vi "MOCON_get_rdg.vi"(4 "Channel Name":string, 7 "Address":T1={"Main"=57344, "Ch."=7, "Sub"=0, "Port Name"="10.245.69.44"}) -> (0 "Output":dbl format="%_5g", 3 "Status note":string)   [LabVIEW 2020]
uses:
  ADAM Client/Sub VIs/ADAM Controls/Address.ctl
  ADAM Client/Sub VIs/ADAM Controls/Remember_value_mode.ctl
panel:
  out "UDPopenError":errorcluster
  out "UDPreadError":errorcluster
  # "Channels:\n0: Timestamp\n1: \n2: \n3: Concentration\n4:\n5:\n6:\n7: Sample Flow\n8: Fuel Flow\n9: Air Flow\n10: Det. Curr.\n11:\n12:\n13: Temperature"
  # "Started life as ClimatronicsUDP_get_rdg.vi"
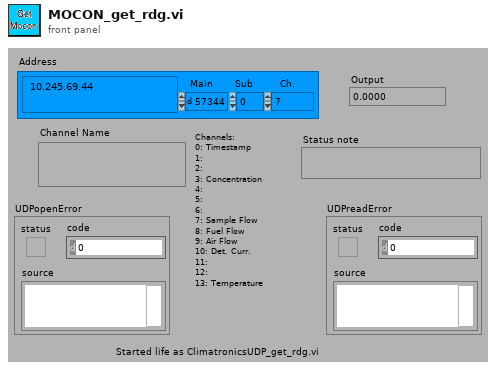
[diagram p1: front panel]
types:
  T1 = typedef "Address.ctl" = cluster{"Main":i32, "Ch.":i32, "Sub":i32, "Port Name":string}
  T2 = typedef "Remember_value_mode.ctl" = enum16{"Read only", "Read and Write"}
  T3 = enum16{"Standard", "Buffered", "CRLF", "Immediate"}
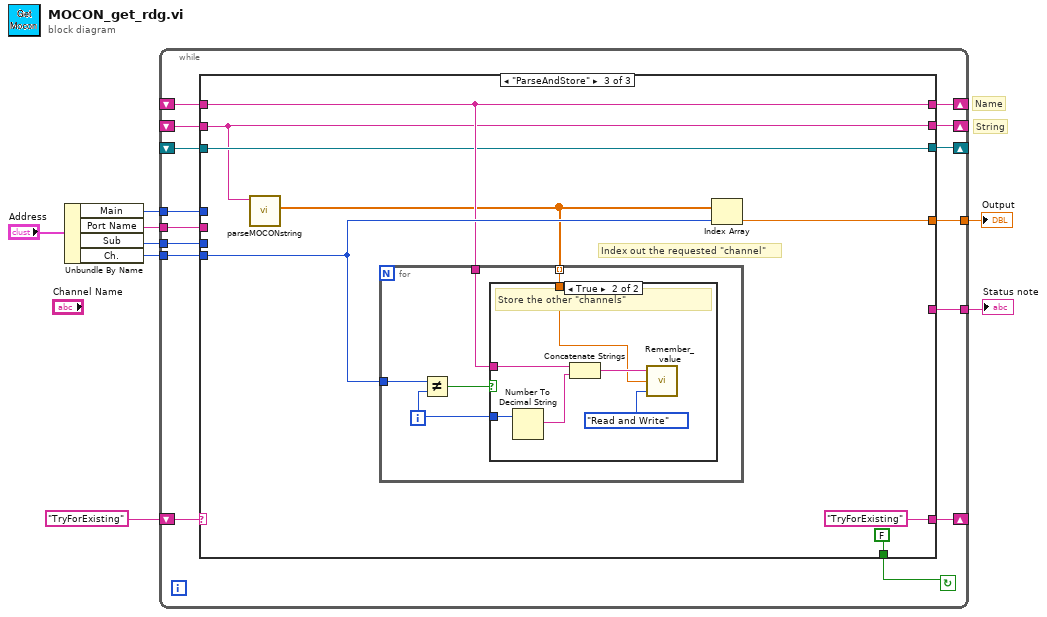
[diagram p0: block diagram]
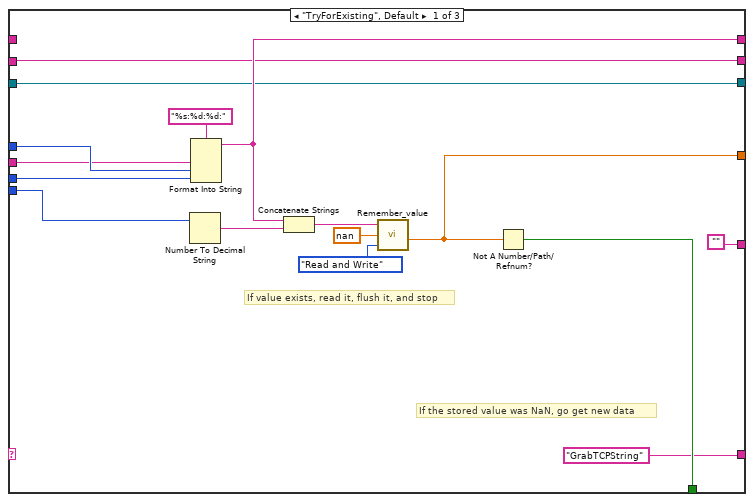
[diagram p2: hidden frame]
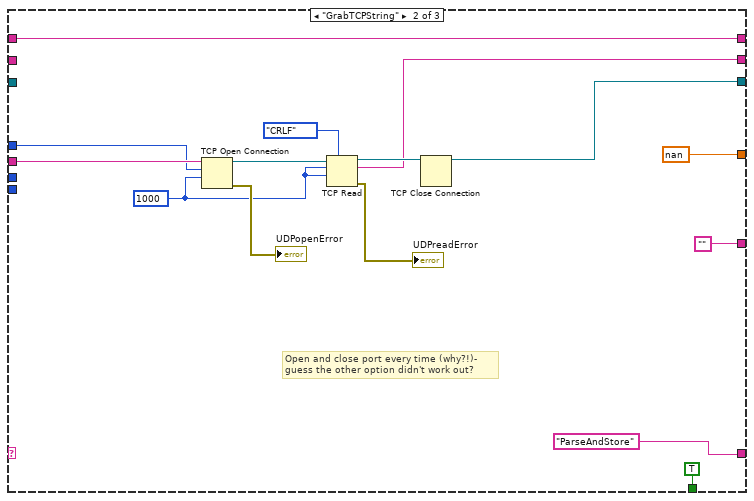
[diagram p3: hidden frame]
diagram:
  # "String"
  # "Name"
  n1 = Unbundle By Name("Address") -> ("Main"=w2:i32, "Port Name"=w7:string, "Sub"=w6:i32, "Ch."=w3:i32)
  n2 = while {
    shift-left: _ -> [w11]
    shift-right: [w12] -> _
    shift-left: _ -> [w14]
    shift-right: [w15] -> _
    tunnel: [w17] -> w4
    tunnel: [w18] -> w5
    shift-left: _ -> [w13]
    shift-right: [w19] -> _
    shift-left: "TryForExisting" -> [w10]
    shift-right: [w9] -> _
    tunnel: w3 -> [w20]
    tunnel: w2 -> [w21]
    tunnel: w6 -> [w22]
    tunnel: w7 -> [w23]
    stop <- w16 continue-if-true
    n3 = case shown="\"ParseAndStore\"" w10 {
      tunnel: w23 -> [w26 w50 _]
      tunnel: w22 -> [w38 _ _]
      tunnel: w21 -> [w39 w41 _]
      tunnel: w20 -> [w36 _ w60]
      tunnel: ["GrabTCPString" "ParseAndStore" "TryForExisting"] -> w9
      tunnel: [w35 w53 w59] -> w19
      tunnel: [w28 nan w61] -> w18
      tunnel: ["" "" _] -> w17
      tunnel: [w27 TRUE FALSE] -> w16
      tunnel: [w30 w46 w56] -> w15
      tunnel: w14 -> [w30 _ w56]
      tunnel: w13 -> [_ w53 w59]
      tunnel: [w25 w43 w58] -> w12
      tunnel: w11 -> [w25 _ w58]
      frame "TryForExisting", Default {
        # "If the stored value was NaN, go get new data"
        # "If value exists, read it, flush it, and stop"
        n4 = Number To Decimal String(number=w36) -> (decimal integer string=w34:string)  [unwired: 1 out]
        n5 = Format Into String(format string="%s:%d:%d:" ("Format String"), w26, w39, w38) -> (resulting string=w35:string)  [unwired: 2 in, 1 out]
        n6 = Concatenate Strings(w35, w34) -> (w33:string)
        n7 = call "Remember_value.vi"("Mode"=Remember_value_mode."Read and Write", "Input Value"=nan, "Ch name"=w33) -> ("Output Value"=w28:dbl)
        n8 = Not A Number/Path/Refnum?(number/path/refnum=w28) -> (NaN/Path/Refnum?=w27:bool)
      }
      frame "GrabTCPString" {
        w40 = 1000 ("timeout ms (60000)")
        # "Open and close port every time (why?!)-\nguess the other option didn't work out?"
        n9 = TCP Open Connection(address=w50, remote port or service name=w41, timeout ms (60000)=w40) -> (connection ID=w49:refnum<k5>, error out=→"UDPopenError":errorcluster)  [unwired: 2 in]
        n10 = TCP Read(connection ID=w49, bytes to read=w40, 7:T3."CRLF" ("mode (standard)"), 9:w40) -> (connection ID out=w47:refnum<k5>, data out=w46:string, error out=→"UDPreadError":errorcluster)  [unwired: 1 in]
        n11 = TCP Close Connection(connection ID=w47) -> (connection ID out=w43:refnum<k5>)  [unwired: 2 in, 1 out]
      }
      frame "ParseAndStore" {
        # "Index out the requested \"channel\""
        n12 = call "parseMOCONstring.vi"("MOCONstring"=w56) -> ("channelsArray"=w55:dbl[])  [unwired: 10 in]
        n13 = for {
          tunnel: w59 -> [w67]
          tunnel: w55 -> [w66] mode=indexing
          tunnel: w60 -> [w64]
          i -> [w65]
          n14 = Not Equal?(x=w64, y=w65) -> (x != y?=w63:bool)
          n15 = case shown="True" w63 {
            tunnel: w65 -> [_ w73]
            tunnel: w67 -> [_ w71]
            tunnel: w66 -> [_ w68]
            frame False {
              # "Don't store the requested channel"
            }
            frame True {
              # "Store the other \"channels\""
              n16 = Number To Decimal String(number=w73) -> (decimal integer string=w72:string)  [unwired: 1 out]
              n17 = Concatenate Strings(w71, w72) -> (w69:string)
              n18 = call "Remember_value.vi"("Mode"=Remember_value_mode."Read and Write", "Input Value"=w68, "Ch name"=w69) -> ()  [unwired: 1 out]
            }
          }
        }
        n19 = Index Array(array=w55, index=w60) -> (element=w61:dbl)
      }
    }
  }
  "Output" <- w5
  "Status note" <- w4
